vi "Handle Error.vi"(8 "error in (no error)":errorcluster, 11 "VDH-VNA_data_handler in":refnum<class "VDH-VNA_data_handler.lvclass">) -> (0 "error out":errorcluster, 2 "stop actor?":bool=TRUE, 3 "VDH-VNA_data_handler out":refnum<class "VDH-VNA_data_handler.lvclass">)   [LabVIEW 2020, in "VDH-VNA_data_handler.lvlib" / "VDH-VNA_data_handler.lvclass"]
doc: "(<B>Filename</B>: Actor Framework.lvlib:Actor.lvclass:Handle Error.vi)\n\nDefines how the actor handles an error that occurred while processing a message. By default, this method does nothing except stop the actor."
uses:
  VDH-VNA_data_handler.lvclass
  <vilib>/ActorFramework/Actor/Actor.lvclass
  common/features/CF-common_features.lvlib
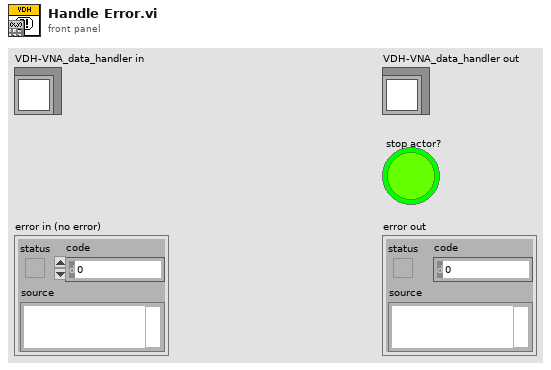
[diagram p1: front panel]
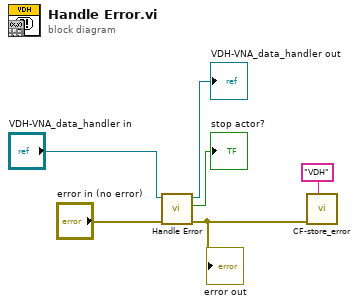
[diagram p0: block diagram]
diagram:
  n1 = call-parent "Handle Error.vi"("error in (no error)"="error in (no error)", "Actor in"="VDH-VNA_data_handler in") -> ("error out"=w1:errorcluster, "stop actor?"=→"stop actor?":bool, "Actor out"=→"VDH-VNA_data_handler out":refnum<class "VDH-VNA_data_handler.lvclass">)  [unwired: 7 in]
  "error out" <- w1
  n2 = call "CF-store_error.vi"("Location"="VDH", "error in (no error)"=w1) -> ()  [unwired: 10 in]
